vi "GetHelp.vi"(11 "RunUnitTests in":refnum<class "RunUnitTests.lvclass">) -> (2 "Help":string, 3 "RunUnitTests out":refnum<class "RunUnitTests.lvclass">)   [LabVIEW 2014, in "RunUnitTests.lvclass"]
uses:
  RunUnitTests.lvclass
panel:
  in  "Help":string="LabVIEWCLI -OperationName RunUnitTests -ProjectPath <path of LabVIEW project> -JUnitReportPath <name of the JUnit report path>]\n\n -ProjectPath : Specifies the full path to the LabVIEW project (.lvproj) file that contains .lvtest files.\n -JUnitReportPath : Specifies the full path to the JUnit report path that will contain test results."
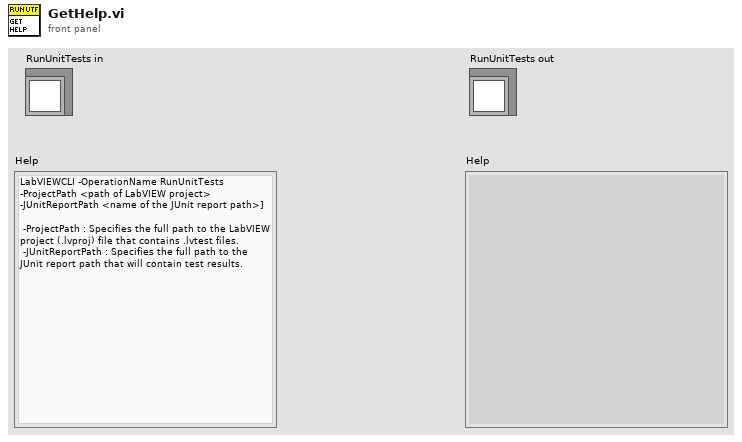
[diagram p1: front panel]
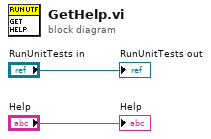
[diagram p0: block diagram]
diagram:
  "RunUnitTests out" <- "RunUnitTests in"
  "Help" <- "Help"
